vi "RPNConversion_Logic.vi"(8 "error in":errorcluster, 10 "Token":string[](array[string]), 11 "Logical Parsed Expression":T1) -> (0 "error out":errorcluster, 3 "Logical Parsed Expression Out":T1)   [LabVIEW 2014, in "SeqLoop.lvlib"]
uses:
  SeqLoop.lvlib
  TypeDefs/LogicParsedExpression.ctl
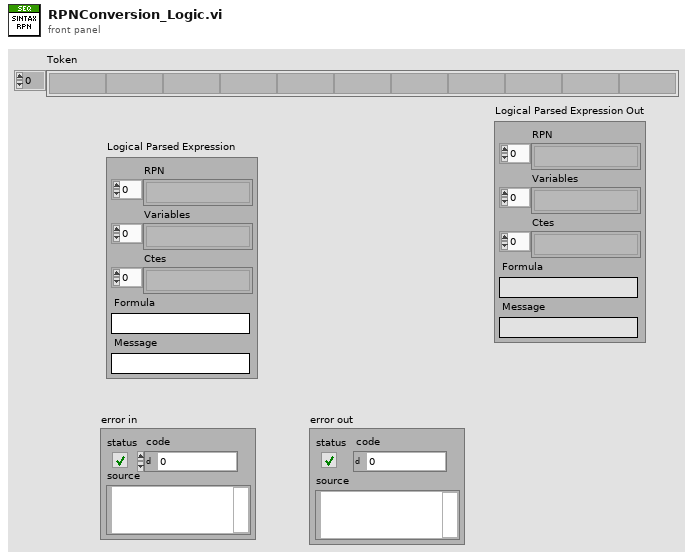
[diagram p1: front panel]
types:
  T1 = typedef "SeqLoop.lvlib/LogicParsedExpression.ctl" = cluster{"RPN ":string[], "Variables":string[], "Ctes":string[], "Formula":string, "Message":string}
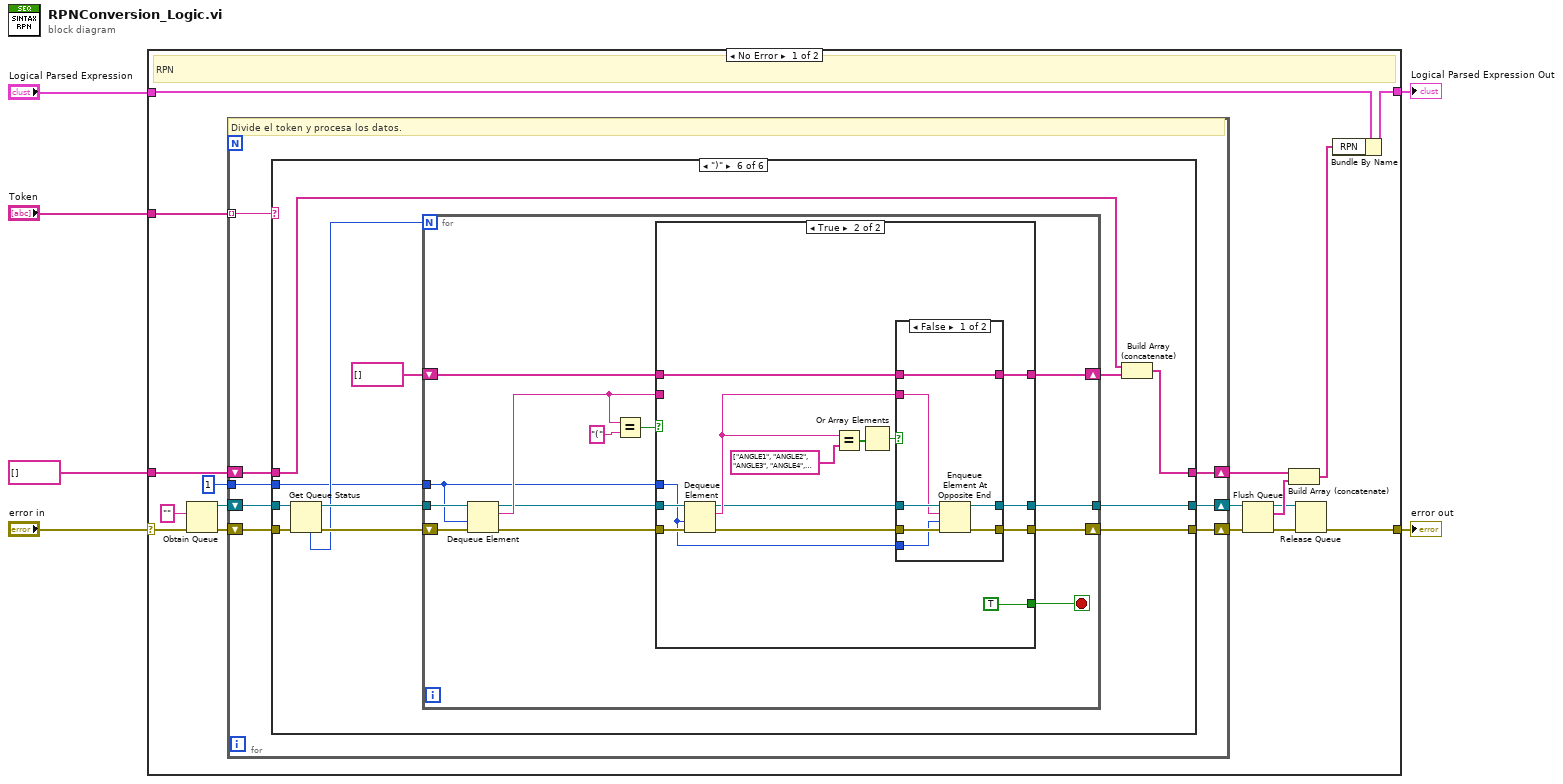
[diagram p0: block diagram]
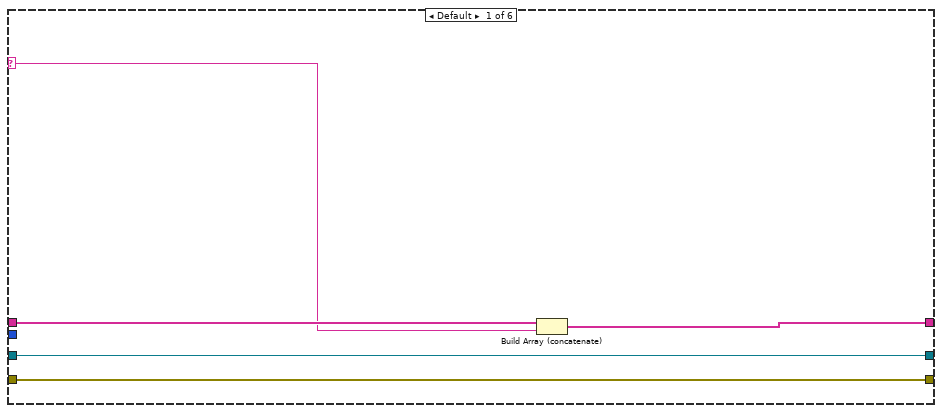
[diagram p2: hidden frame]
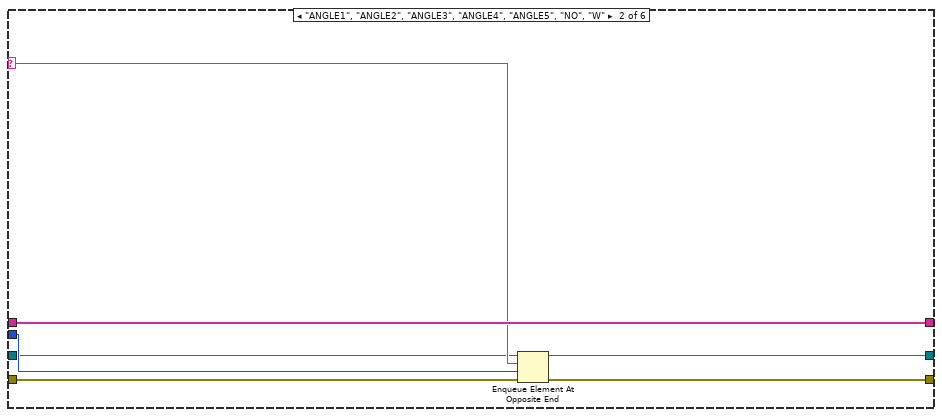
[diagram p3: hidden frame]
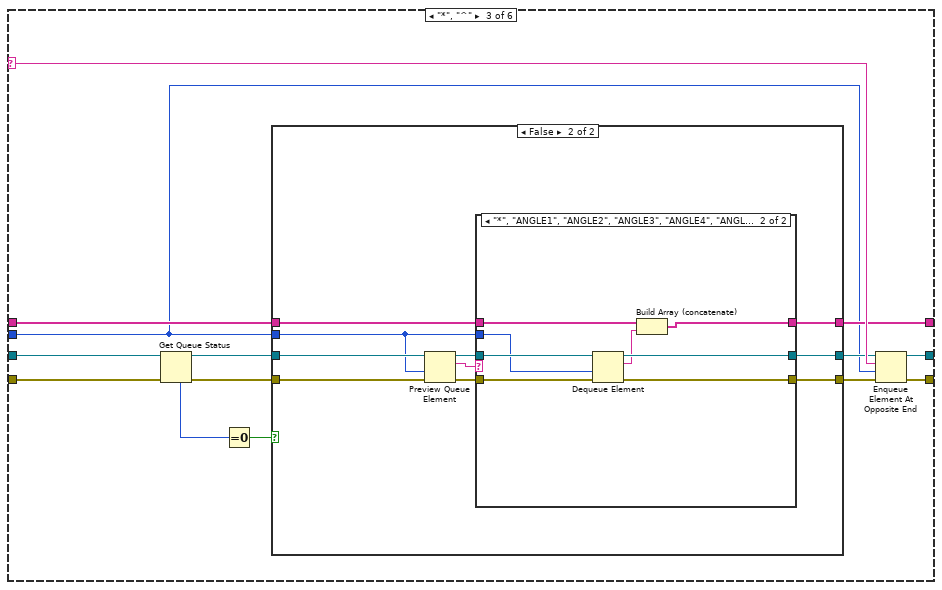
[diagram p4: hidden frame]
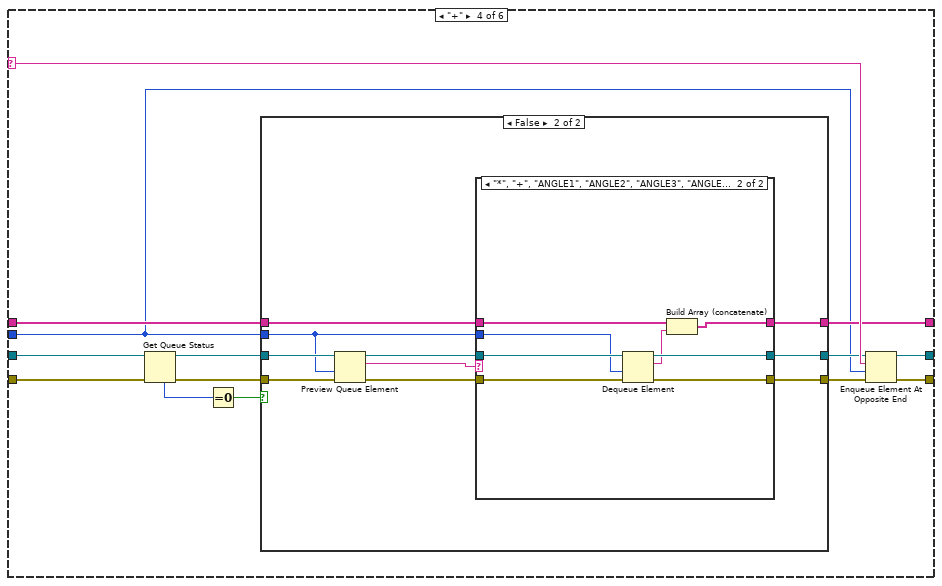
[diagram p7: hidden frame]
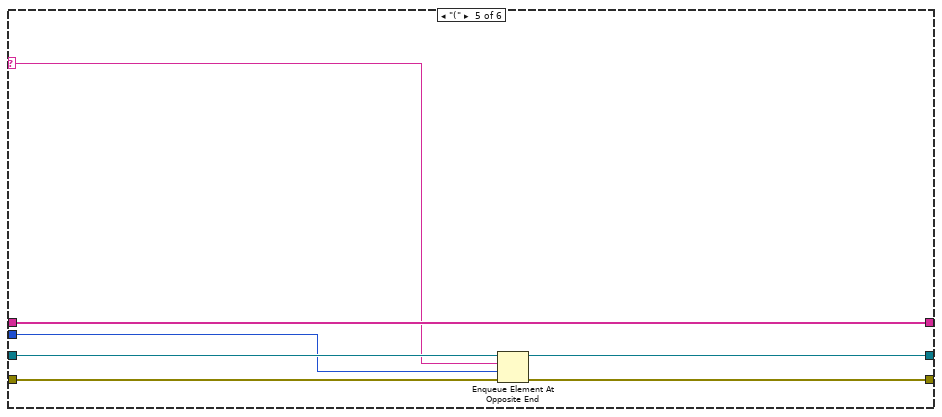
[diagram p10: hidden frame]
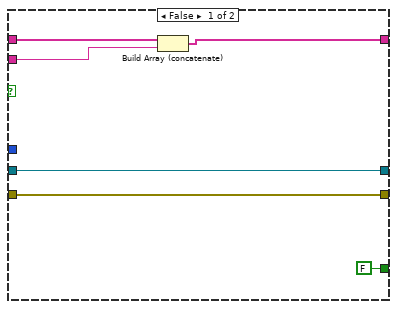
[diagram p11: hidden frame]
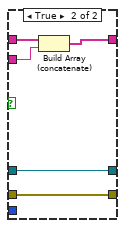
[diagram p12: hidden frame]
diagram:
  n1 = case shown="No Error" "error in" {
    selector: "error in" -> [w10 w184]
    tunnel: [w14 w184] -> w6
    tunnel: "Token" -> [w12 _]
    tunnel: string[] [] -> [w11 _]
    tunnel: "Logical Parsed Expression" -> [w9 w185]
    tunnel: [w8 w185] -> w2
    frame No Error {
      # "RPN"
      n2 = Obtain Queue(element data type="", error in (no error)=w10) -> (queue out=w13:refnum<queue>, error out=w23:errorcluster)  [unwired: 3 in, 1 out]
      n3 = for {
        tunnel: w12 -> [w31] mode=indexing
        shift-right: [w28] -> w21
        shift-left: w13 -> [w30]
        shift-right: [w27] -> w20
        shift-left: w23 -> [w29]
        shift-right: [w25] -> w19
        shift-left: w11 -> [w26]
        tunnel: 1 -> [w24]
        # "Divide el token y procesa los datos."
        n4 = case shown="\")\"" w31 {
          selector: w31 -> [w35 w40 w55 w93 w121 _]
          tunnel: w30 -> [w33 w38 w54 w92 w126 w138]
          tunnel: w29 -> [w32 w37 w48 w86 w125 w136]
          tunnel: [w33 w42 w57 w95 w124 w129] -> w28
          tunnel: [w32 w43 w56 w94 w123 w128] -> w27
          tunnel: w26 -> [w36 w41 w51 w89 w122 w133]
          tunnel: [w34 w41 w50 w88 w122 w132] -> w25
          tunnel: w24 -> [_ w39 w44 w82 w120 w130]
          frame Default {
            n5 = Build Array (concatenate)(w36, w35) -> (w34:string[])
          }
          frame "ANGLE1", "ANGLE2", "ANGLE3", "ANGLE4", "ANGLE5", "NO", "W" {
            n6 = Enqueue Element At Opposite End(queue=w38, element=w40, timeout in ms (-1)=w39, error in (no error)=w37) -> (queue out=w42:refnum<queue>, error out=w43:errorcluster)  [unwired: 1 out]
          }
          frame "*", "^" {
            n7 = Get Queue Status(queue=w54, error in (no error)=w48) -> (queue out=w49:refnum<queue>, error out=w47:errorcluster, # elements in queue=w45:i32)  [unwired: 1 in, 5 out]
            n8 = Equal To 0?(x=w45) -> (x = 0?=w46:bool)
            n9 = case shown="False" w46 {
              tunnel: w49 -> [w59 w70]
              tunnel: w47 -> [w58 w69]
              tunnel: [w59 w65] -> w53
              tunnel: [w58 w64] -> w52
              tunnel: w51 -> [w60 w63]
              tunnel: [w60 w62] -> w50
              tunnel: w44 -> [_ w61]
              frame True {
              }
              frame False {
                n10 = Preview Queue Element(queue=w70, timeout in ms (-1)=w61, error in (no error)=w69) -> (queue out=w67:refnum<queue>, element=w68:string, error out=w66:errorcluster)  [unwired: 1 out]
                n11 = case shown="\"*\", \"ANGLE1\", \"ANGLE2\", \"ANGLE3\", \"ANGLE4\", \"ANGLE5\", \"NO\", \"W\", \"^\"" w68 {
                  tunnel: w67 -> [w73 w81]
                  tunnel: w66 -> [w72 w80]
                  tunnel: [w73 w79] -> w65
                  tunnel: [w72 w78] -> w64
                  tunnel: w63 -> [w71 w77]
                  tunnel: [w71 w75] -> w62
                  tunnel: w61 -> [_ w74]
                  frame Default {
                  }
                  frame "*", "ANGLE1", "ANGLE2", "ANGLE3", "ANGLE4", "ANGLE5", "NO", "W", "^" {
                    n12 = Dequeue Element(queue=w81, timeout in ms (-1)=w74, error in (no error)=w80) -> (queue out=w79:refnum<queue>, element=w76:string, error out=w78:errorcluster)  [unwired: 1 out]
                    n13 = Build Array (concatenate)(w77, w76) -> (w75:string[])
                  }
                }
              }
            }
            n14 = Enqueue Element At Opposite End(queue=w53, element=w55, timeout in ms (-1)=w44, error in (no error)=w52) -> (queue out=w57:refnum<queue>, error out=w56:errorcluster)  [unwired: 1 out]
          }
          frame "+" {
            n15 = Get Queue Status(queue=w92, error in (no error)=w86) -> (queue out=w87:refnum<queue>, error out=w85:errorcluster, # elements in queue=w83:i32)  [unwired: 1 in, 5 out]
            n16 = Equal To 0?(x=w83) -> (x = 0?=w84:bool)
            n17 = case shown="False" w84 {
              tunnel: w87 -> [w97 w108]
              tunnel: w85 -> [w96 w107]
              tunnel: [w97 w103] -> w91
              tunnel: [w96 w102] -> w90
              tunnel: w89 -> [w98 w101]
              tunnel: [w98 w100] -> w88
              tunnel: w82 -> [_ w99]
              frame True {
              }
              frame False {
                n18 = Preview Queue Element(queue=w108, timeout in ms (-1)=w99, error in (no error)=w107) -> (queue out=w105:refnum<queue>, element=w106:string, error out=w104:errorcluster)  [unwired: 1 out]
                n19 = case shown="\"*\", \"+\", \"ANGLE1\", \"ANGLE2\", \"ANGLE3\", \"ANGLE4\", \"ANGLE5\", \"NO\", \"W\", \"^\"" w106 {
                  tunnel: w105 -> [w111 w119]
                  tunnel: w104 -> [w110 w118]
                  tunnel: [w111 w117] -> w103
                  tunnel: [w110 w116] -> w102
                  tunnel: w101 -> [w109 w115]
                  tunnel: [w109 w113] -> w100
                  tunnel: w99 -> [_ w112]
                  frame Default {
                  }
                  frame "*", "+", "ANGLE1", "ANGLE2", "ANGLE3", "ANGLE4", "ANGLE5", "NO", "W", "^" {
                    n20 = Dequeue Element(queue=w119, timeout in ms (-1)=w112, error in (no error)=w118) -> (queue out=w117:refnum<queue>, element=w114:string, error out=w116:errorcluster)  [unwired: 1 out]
                    n21 = Build Array (concatenate)(w115, w114) -> (w113:string[])
                  }
                }
              }
            }
            n22 = Enqueue Element At Opposite End(queue=w91, element=w93, timeout in ms (-1)=w82, error in (no error)=w90) -> (queue out=w95:refnum<queue>, error out=w94:errorcluster)  [unwired: 1 out]
          }
          frame "(" {
            n23 = Enqueue Element At Opposite End(queue=w126, element=w121, timeout in ms (-1)=w120, error in (no error)=w125) -> (queue out=w124:refnum<queue>, error out=w123:errorcluster)  [unwired: 1 out]
          }
          frame ")" {
            n24 = Get Queue Status(queue=w138, error in (no error)=w136) -> (queue out=w137:refnum<queue>, error out=w135:errorcluster, # elements in queue=w134:i32)  [unwired: 1 in, 5 out]
            n25 = for {
              N: w134 -> [_]
              tunnel: w137 -> [w151]
              tunnel: [w146] -> w129
              shift-right: [w144] -> w128
              shift-left: w135 -> [w150]
              tunnel: w130 -> [w142]
              shift-right: [w148] -> w127
              shift-left: string[] [] ("Array") -> [w149]
              stop <- w139 stop-if-true
              n26 = Dequeue Element(queue=w151, timeout in ms (-1)=w142, error in (no error)=w150) -> (queue out=w145:refnum<queue>, element=w147:string, error out=w143:errorcluster)  [unwired: 1 out]
              n27 = Equal?(x=w147, y="(") -> (x = y?=w140:bool)
              n28 = case shown="True" w140 {
                tunnel: w149 -> [w156 w170]
                tunnel: w147 -> [w157 _]
                tunnel: [w155 w171] -> w148
                tunnel: [w154 w163] -> w146
                tunnel: w145 -> [w154 w169]
                tunnel: [w153 w162] -> w144
                tunnel: w143 -> [w153 w168]
                tunnel: w142 -> [_ w159]
                tunnel: [FALSE TRUE] -> w139
                frame False {
                  n29 = Build Array (concatenate)(w156, w157) -> (w155:string[])
                }
                frame True {
                  n30 = Dequeue Element(queue=w169, timeout in ms (-1)=w159, error in (no error)=w168) -> (queue out=w161:refnum<queue>, element=w166:string, error out=w160:errorcluster)  [unwired: 1 out]
                  n31 = Equal?(x=w166, y=string[] ["ANGLE1", "ANGLE2", "ANGLE3", "ANGLE4", "ANGLE5", "NO", "W"] ("Funciones")) -> (x = y?=w167:bool[])
                  n32 = Or Array Elements(Boolean array=w167) -> (logical OR=w165:bool)
                  n33 = case shown="False" w165 {
                    tunnel: [w178 w183] -> w171
                    tunnel: w170 -> [w178 w182]
                    tunnel: w166 -> [w173 w181]
                    tunnel: [w177 w180] -> w163
                    tunnel: [w176 w179] -> w162
                    tunnel: w161 -> [w175 w180]
                    tunnel: w160 -> [w174 w179]
                    tunnel: w159 -> [w172 _]
                    frame False {
                      n34 = Enqueue Element At Opposite End(queue=w175, element=w173, timeout in ms (-1)=w172, error in (no error)=w174) -> (queue out=w177:refnum<queue>, error out=w176:errorcluster)  [unwired: 1 out]
                    }
                    frame True {
                      n35 = Build Array (concatenate)(w182, w181) -> (w183:string[])
                    }
                  }
                }
              }
            }
            n36 = Build Array (concatenate)(w133, w127) -> (w132:string[])
          }
        }
      }
      n37 = Flush Queue(queue=w21, error in (no error)=w20) -> (queue out=w17:refnum<queue>, remaining elements=w18:string[], error out=w16:errorcluster)
      n38 = Build Array (concatenate)(w19, w18) -> (w7:string[])
      n39 = Release Queue(queue=w17, error in (no error)=w16) -> (error out=w14:errorcluster)  [unwired: 1 in, 2 out]
      n40 = Bundle By Name(cluster=w9, "RPN"=w7) -> (w8:T1)
    }
    frame Error {
    }
  }
  "error out" <- w6
  "Logical Parsed Expression Out" <- w2
